vi "Read Subpanels.vi"(8 "error in (no error)":errorcluster, 11 "Application in":refnum<class "Application.lvclass">) -> (0 "error out":errorcluster, 2 "Subpanels":T1, 3 "Application out":refnum<class "Application.lvclass">)   [LabVIEW 2016, in "Application.lvclass"]
uses:
  Application.lvclass
  FrontPanelControls.ctl
  Application.lvclass/Application.ctl
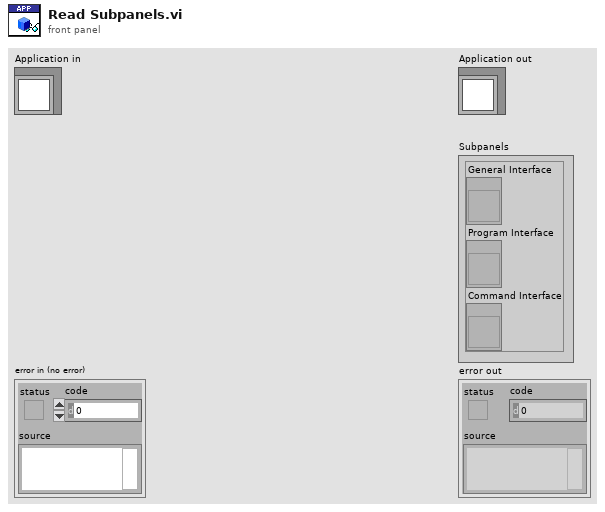
[diagram p1: front panel]
types:
  T1 = typedef "Application.lvclass/FrontPanelControls.ctl" = cluster{"General Interface":refnum<vi>, "Program Interface":refnum<vi>, "Command Interface":refnum<vi>}
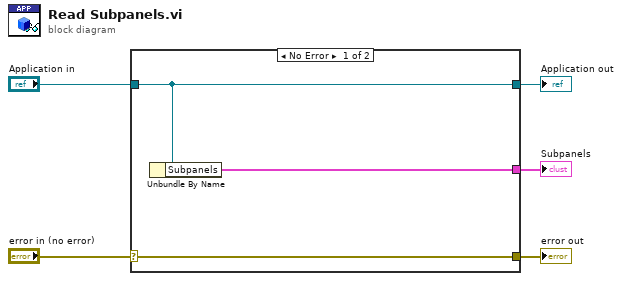
[diagram p0: block diagram]
diagram:
  n1 = case shown="No Error" "error in (no error)" {
    selector: "error in (no error)" -> [w8 w9]
    tunnel: [w8 w9] -> w4
    tunnel: [w7 w10] -> w2
    tunnel: "Application in" -> [w7 w10]
    tunnel: [w6 _] -> w1
    frame No Error {
      n2 = Unbundle By Name(w7) -> ("Subpanels"=w6:T1)
    }
    frame Error {
    }
  }
  "error out" <- w4
  "Application out" <- w2
  "Subpanels" <- w1
